vi "TEST STEER.vi"() -> ()   [LabVIEW 2023]
uses:
  ctrl defs/ctrl MOTOR SELECT.ctl
  <vilib>/Rock Robotics/WPI/ThirdParty/REV Robotics/REVLib/Typedef/Spark MAX Idle Mode.ctl
  ctrl defs/ctrl swerve motor.ctl
  ctrl defs/ctrl Spark MAX current limiting.ctl
  ctrl defs/ctrl motor PIDF coefficients.ctl
  <vilib>/Rock Robotics/WPI/ThirdParty/REV Robotics/REVLib/Typedef/Spark MAX Smart Motion Parameters.ctl
  <vilib>/Rock Robotics/WPI/MotorControl/WPI_MotorControlDeviceRef.ctl
  <vilib>/Rock Robotics/WPI/MotorControl/WPI_MotorControlType.ctl
  <vilib>/Rock Robotics/SystemInterfaces/DIO/FPGA_DIOPWMChannel.ctl
  <vilib>/Rock Robotics/WPI/PWM/WPI_PWMDeadband.ctl
  <vilib>/Rock Robotics/SystemInterfaces/DIO/FPGA_DIOChannel.ctl
  <vilib>/Rock Robotics/WPI/ThirdParty/Phoenix-LabVIEW/CANCoder/Controls/CTRE_Phoenix_CANcoder_DeviceRef.ctl
  <vilib>/Rock Robotics/WPI/ThirdParty/REV Robotics/REVLib/Typedef/Spark MAX Control Type.ctl
  Global INIT.vi
  <vilib>/Rock Robotics/WPI/ThirdParty/Phoenix-LabVIEW/CANCoder/Get/CTRE_Phoenix_CANcoder_GetSensorData.vi
panel:
  out "Absolute Position":dbl
  out "Velocity":dbl
  out "Position":dbl
  in  "Magnet Offset (Degrees)":dbl
  in  "Sensor Direction":bool
  in  "refnum name 2":string
  in  "CAN Bus":string
  in  "CAN ID 2":u8
  in  "Installed? 2":bool
  in  "description 2":string
  out "Sensor Velocity":dbl
  out "Sensor Position":dbl
  out "Hard Limit Rev":bool
  out "Hard Limit Fwd":bool
  in  "MOTOR %VBus":dbl(slide) scale=-1.0..1.0
  out "swerve STEER motors":T1[](array[typedef]) {"gear ratio" format="%_5f"; "MOTOR SELECT" items=["REV NEO"=5676, "REV NEO 550"=11000, "VEX Falcon"=6380, "WC Kraken"=6000]}
  in  "SAFETY":bool
  in  "commit to INIT":bool
  in  "commit WRITE":bool
  in  "Idle Mode":T3
  in  "Invert":bool
  in  "refnum name":string
  in  "CAN ID":u8
  in  "Installed?":bool
  in  "MOTOR SELECT":T2 items=["REV NEO"=5676, "REV NEO 550"=11000, "VEX Falcon"=6380, "WC Kraken"=6000]
  in  "description":string
  in  "stop":bool
  in  "Select\nSTEER motor":T7(ring)=enum."Front Left"
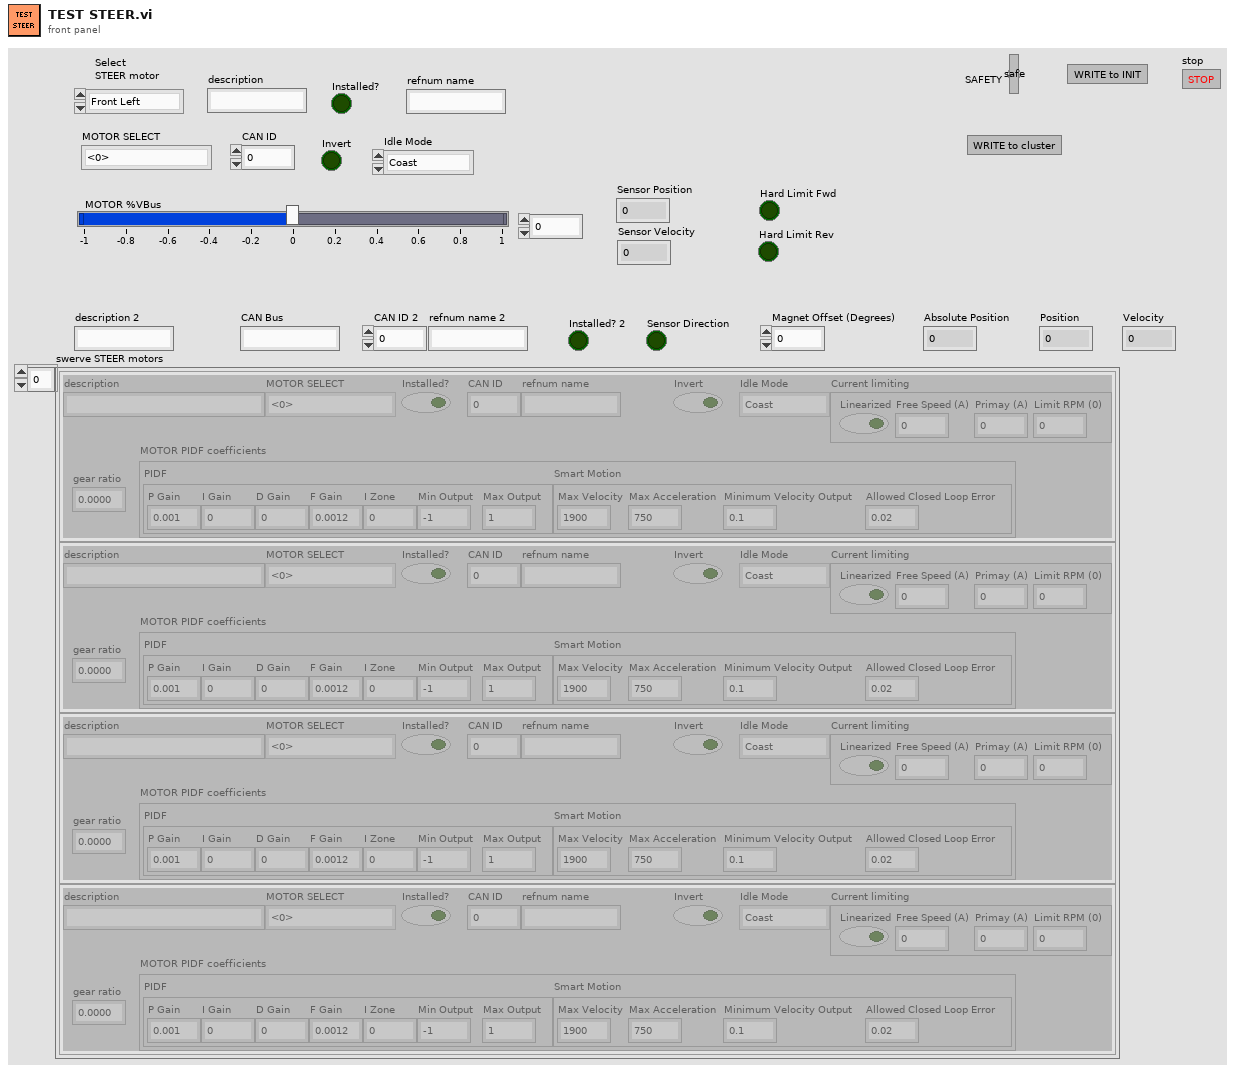
[diagram p1: front panel]
types:
  T1 = typedef "ctrl swerve motor.ctl" = cluster{"description":string, "MOTOR SELECT":T2, "Installed?":bool, "CAN ID":u8, "refnum name":string, "Invert":bool, "Idle Mode":T3, "Current limiting":T4, "MOTOR PIDF coefficients":T5, "gear ratio":dbl}
  T2 = typedef "ctrl MOTOR SELECT.ctl" = i16
  T3 = typedef "Spark MAX Idle Mode.ctl" = enum16{"Coast", "Brake"}
  T4 = typedef "ctrl Spark MAX current limiting.ctl" = cluster{"Linearized":bool, "Free Speed (A)":dbl, "Primay (A)":dbl, "Limit RPM (0)":u32}
  T5 = typedef "ctrl motor PIDF coefficients.ctl" = cluster{"PIDF":cluster{"P Gain":dbl, "I Gain":dbl, "D Gain":dbl, "F Gain":dbl, "I Zone":dbl, "Min Output":dbl, "Max Output":dbl}, "Smart Motion":T6}
  T6 = typedef "Spark MAX Smart Motion Parameters.ctl" = cluster{"Max Velocity":dbl, "Max Acceleration":dbl, "Minimum Velocity Output":dbl, "Allowed Closed Loop Error":dbl}
  T7 = enum16{"Front Right", "Front Left", "Rear Left", "Rear Right"}
  T8 = typedef "CTRE_Phoenix_CANcoder_DeviceRef.ctl" = cluster{"DeviceStatus":errorcluster, "Device Number":u8, "Handle":u64, "UsageFrame":u32, "Library Path":path}
  T9 = typedef "WPI_MotorControlDeviceRef.ctl" = cluster{"DeviceStatus":errorcluster, "Type":T10, "PWM":cluster{"PWM Channel":T11, "DeadBand":T12}, "CAN":cluster{"Device Number":u8, "SetOutput VI Ref":variant, "GetOutput VI Ref":variant, "Enable VI Ref":variant, "Disable VI Ref":variant, "Data":variant}, "Invert":bool, "DIO PWM":cluster{"PWM \"Enable\" Channel":T11, "DIOChannel":T13, "PWM Rate":dbl}}
  T10 = typedef "WPI_MotorControlType.ctl" = enum16{"PWM", "CAN", "DIO PWM"}
  T11 = typedef "FPGA_DIOPWMChannel.ctl" = enum8{"PWM 0", "PWM 1", "PWM 2", "PWM 3", "PWM 4", "PWM 5", "PWM 6", "PWM 7", "PWM 8", "PWM 9", "PWM MXP 0", "PWM MXP 1", "PWM MXP 2", "PWM MXP 3", "PWM MXP 4", "PWM MXP 5", "PWM MXP 6", "PWM MXP 7", "PWM MXP 8", "PWM MXP 9", "Invalid"}
  T12 = typedef "WPI_PWMDeadband.ctl" = cluster{"Name":string, "maxPositivePwm":i32, "minPositivePwm":i32, "centerPwm":i32, "maxNegativePwm":i32, "minNegativePwm":i32, "angularRange":u16}
  T13 = typedef "FPGA_DIOChannel.ctl" = enum8{"DIO 0", "DIO 1", "DIO 2", "DIO 3", "DIO 4", "DIO 5", "DIO 6", "DIO 7", "DIO 8", "DIO 9", "DIO MXP 0", "DIO MXP 1", "DIO MXP 2", "DIO MXP 3", "DIO MXP 4", "DIO MXP 5", "DIO MXP 6", "DIO MXP 7", "DIO MXP 8", "DIO MXP 9", "DIO MXP 10", "DIO MXP 11", "DIO MXP 12", "DIO MXP 13", "DIO MXP 14", "DIO MXP 15", "SPI Port CS1", "SPI Port CS2", "SPI Port CS3", "SPI Port MISO", "SPI Port MOSI", "Invalid"}
  T14 = typedef "ctrl CANcoder.ctl" = cluster{"description":string, "Installed?":bool, "CAN ID":u8, "CAN Bus":string, "refnum name":string, "Sensor Direction":bool, "Magnet Offset (Degrees)":dbl, "gear ratio":dbl}
  T15 = typedef "Spark MAX Control Type.ctl" = enum16{"Percent VBus", "Voltage", "Velocity", "Position", "Smart Motion", "Current", "Smart Velocity"}
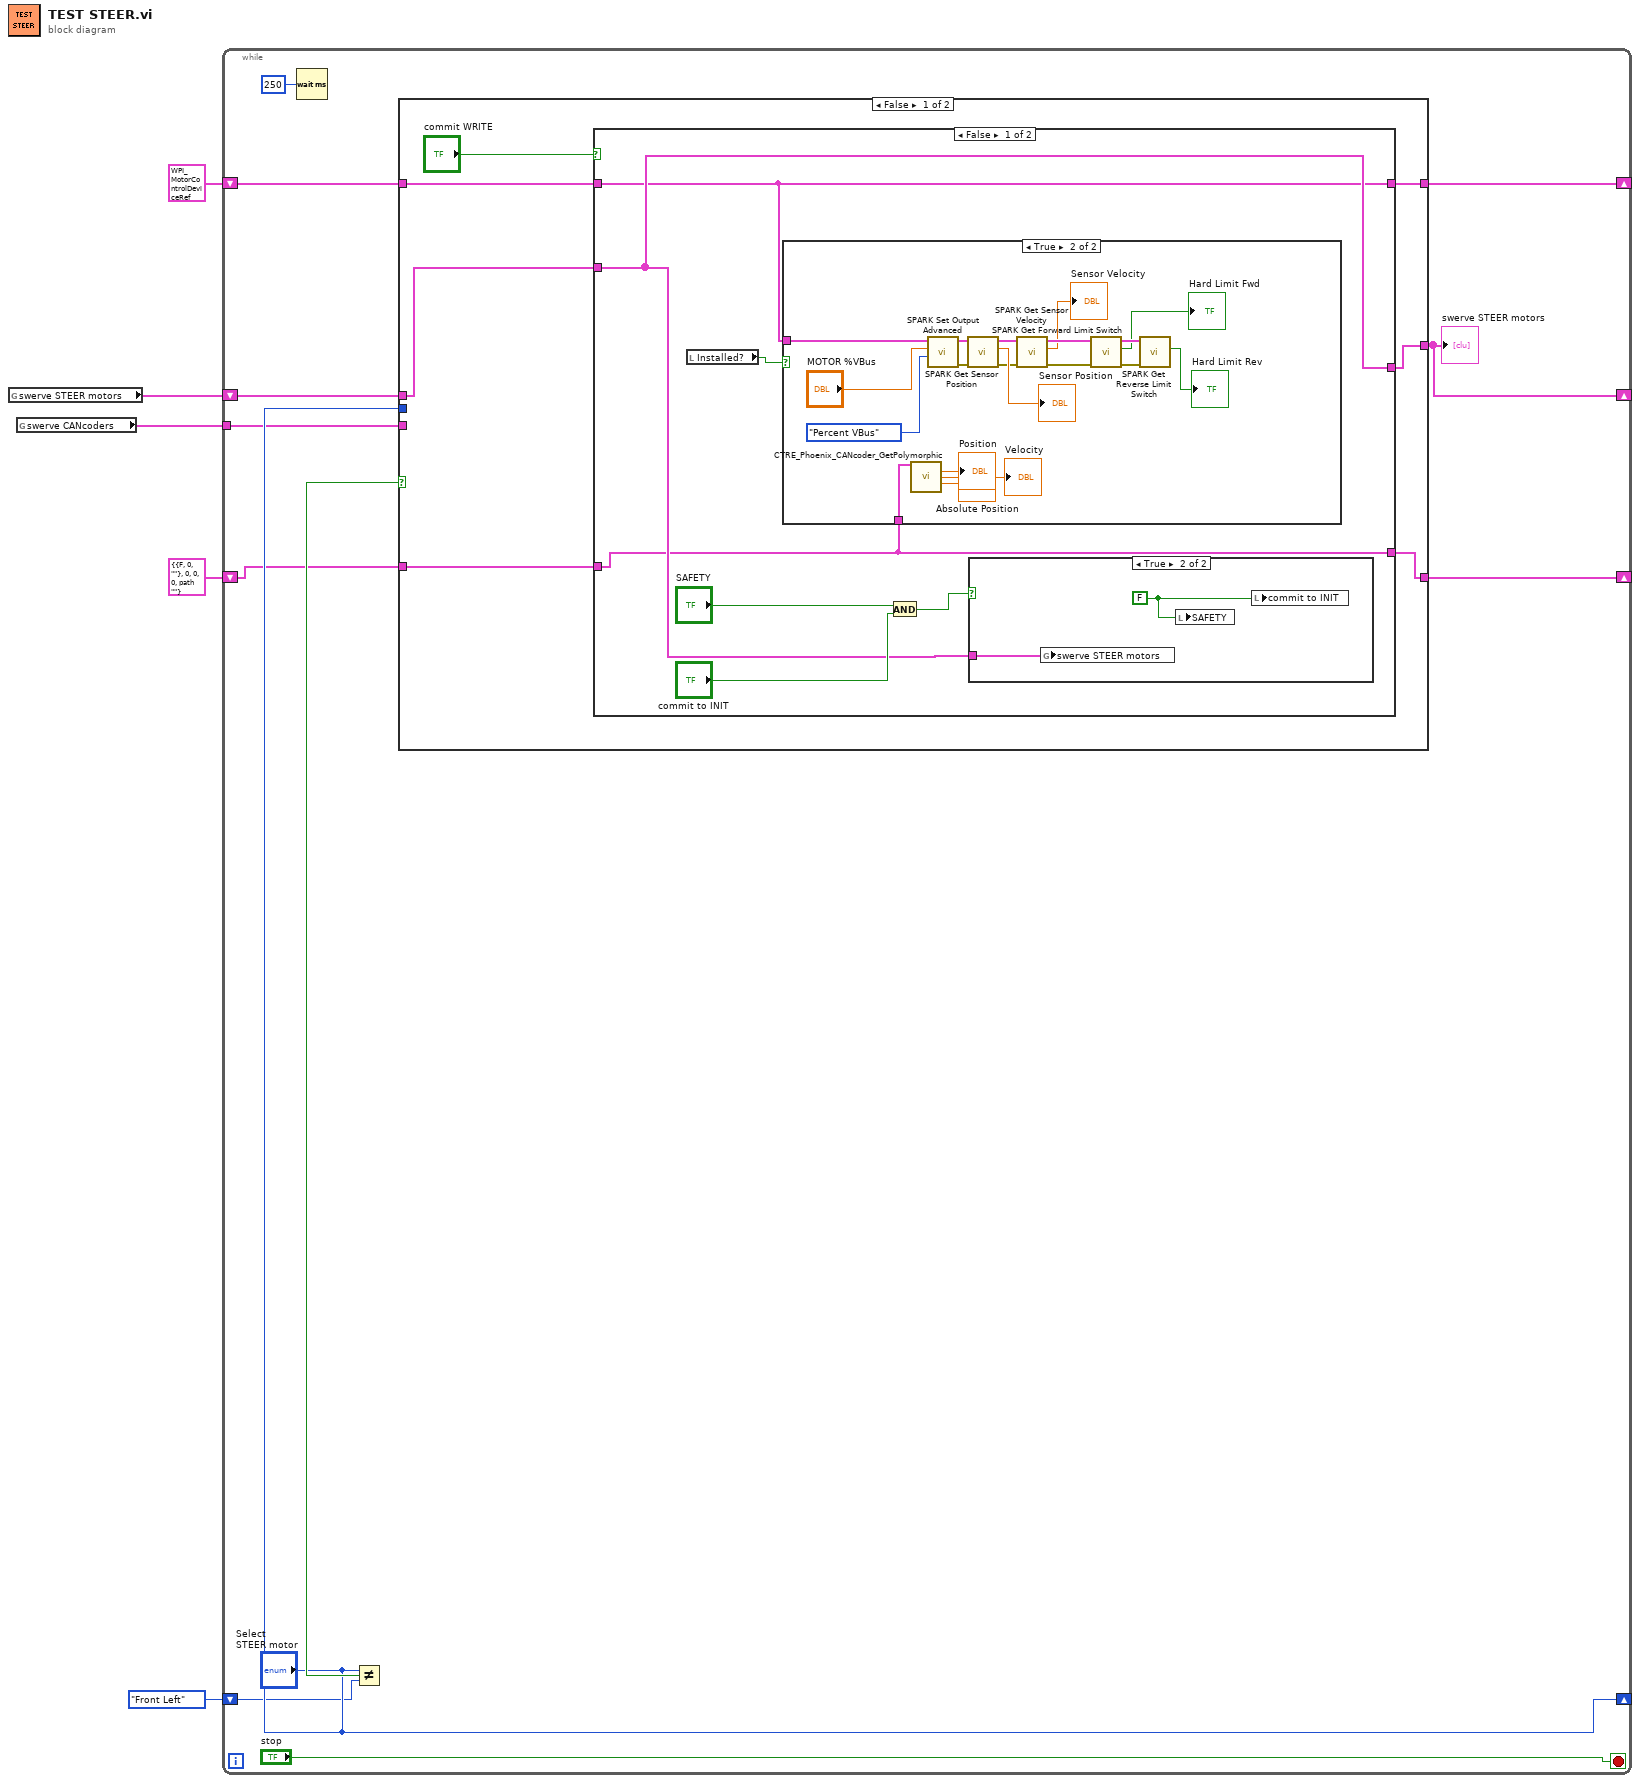
[diagram p0: block diagram]
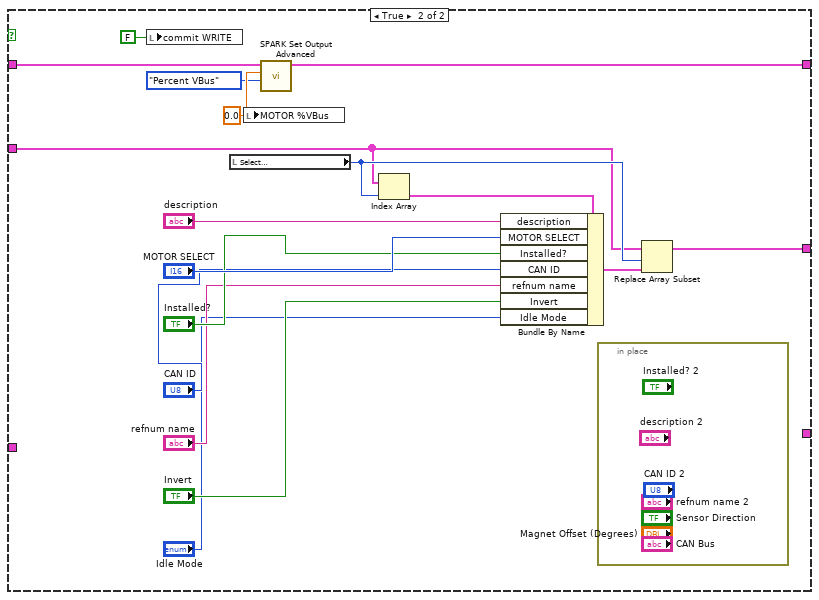
[diagram p4: hidden frame]
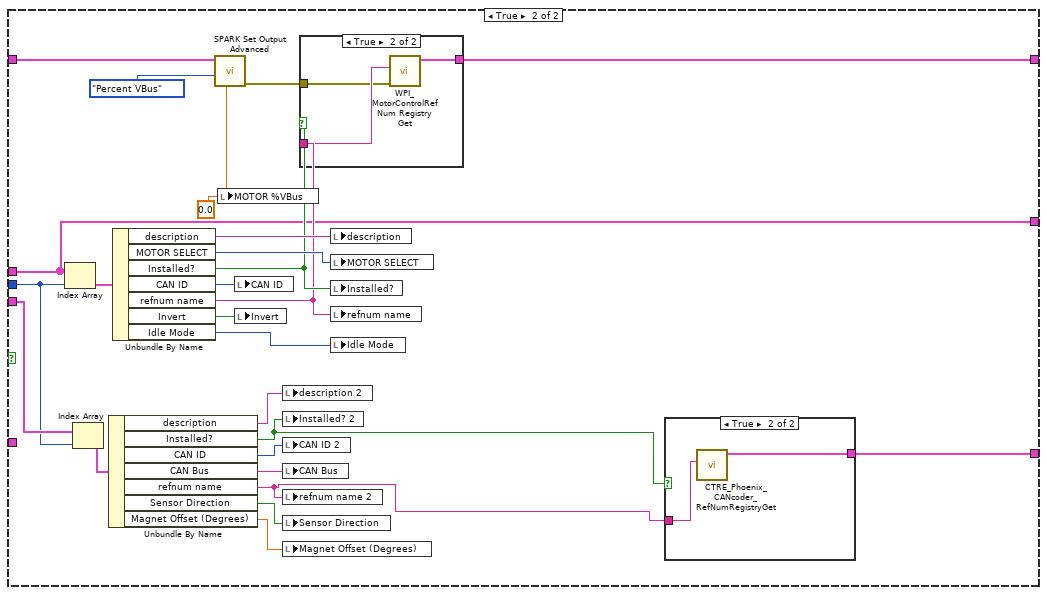
[diagram p5: hidden frame]
diagram:
  n1 = global read "Global INIT.vi" "swerve STEER motors"() -> (w5:T1[])
  n2 = global read "Global INIT.vi" "swerve CANcoders"() -> (w2:T14[])
  n3 = while {
    shift-right: ["Select\nSTEER motor"] -> _
    shift-left: T7."Front Left" ("Select\nSTEER motor") -> [w14]
    shift-right: [w12] -> _
    shift-left: w5 -> [w13]
    shift-right: [w10] -> _
    shift-left: T9 {"DeviceStatus"={"status"=FALSE, "code"=0, "source"=""}, "Type"=enum."PWM", "PWM"={"PWM Channel"=enum."Invalid", "DeadBand"={"Name"="", "maxPositivePwm"=0, "minPositivePwm"=0, "centerPwm"=0, "maxNegativePwm"=0, "minNegativePwm"=0, "angularRange"=0}}, "CAN"={"Device Number"=0, "SetOutput VI Ref"=variant, "GetOutput VI Ref"=variant, "Enable VI Ref"=variant, "Disable VI Ref"=variant, "Data"=variant}, "Invert"=FALSE, "DIO PWM"={"PWM \"Enable\" Channel"=enum."Invalid", "DIOChannel"=enum."Invalid", "PWM Rate"=0.0}} ("MotorControlDevRef") -> [w9]
    tunnel: w2 -> [w8]
    shift-right: [w7] -> _
    shift-left: T8 {"DeviceStatus"={"status"=FALSE, "code"=0, "source"=""}, "Device Number"=0, "Handle"=0, "UsageFrame"=0, "Library Path"=path ""} ("CTRE_CANcoder_DeviceRef") -> [w6]
    stop <- "stop" stop-if-true
    n4 = Wait (ms)(milliseconds to wait=u32 250) -> ()  [unwired: 1 out]
    n5 = Not Equal?(x="Select\nSTEER motor", y=w14) -> (x != y?=w16:bool)
    n6 = case shown="False" w16 {
      tunnel: w13 -> [w20 w81]
      tunnel: "Select\nSTEER motor" -> [_ w79]
      tunnel: [w23 w81] -> w12
      tunnel: [w21 w86] -> w10
      tunnel: w9 -> [w22 w83]
      tunnel: w8 -> [_ w80]
      tunnel: [w18 w77] -> w7
      tunnel: w6 -> [w19 _]
      frame False {
        n7 = case shown="False" "commit WRITE" {
          tunnel: w20 -> [w28 w66]
          tunnel: [w28 w68] -> w23
          tunnel: w22 -> [w25 w56]
          tunnel: [w25 w55] -> w21
          tunnel: w19 -> [w26 _]
          tunnel: [w26 _] -> w18
          frame False {
            n8 = local read "Installed?"() -> (w27:bool)
            n9 = case shown="True" w27 {
              tunnel: w25 -> [_ w50]
              tunnel: w26 -> [_ w35]
              frame False {
              }
              frame True {
                n10 = call-poly <vilib>:"CTRE_Phoenix_CANcoder_GetPolymorphic.vi"("CTRE_CANcoder_DeviceRef"=w35) -> ("Position"=→"Position":dbl, "Velocity"=→"Velocity":dbl, "Absolute Position"=→"Absolute Position":dbl)  [unwired: 10 in, 2 out]
                n11 = call <vilib>:"SPARK Set Output Advanced.vi"("Control Mode"=Spark_MAX_Control_Type."Percent VBus", "Setpoint"="MOTOR %VBus", "MotorControlDevRef"=w50) -> ("error out"=w40:errorcluster, "MotorControlDevRef"=w41:T9)  [unwired: 7 in]
                n12 = call <vilib>:"SPARK Get Sensor Position.vi"("error in (no error)"=w40, "MotorControlDevRef in"=w41) -> ("error out"=w43:errorcluster, "Sensor Position"=→"Sensor Position":dbl, "MotorControlDevRef out"=w47:T9)  [unwired: 6 in, 1 out]
                n13 = call <vilib>:"SPARK Get Sensor Velocity.vi"("error in (no error)"=w43, "MotorControlDevRef in"=w47) -> ("error out"=w42:errorcluster, "Sensor Velocity"=→"Sensor Velocity":dbl, "MotorControlDevRef out"=w46:T9)  [unwired: 6 in, 1 out]
                n14 = call <vilib>:"SPARK Get Forward Limit Switch.vi"("error in (no error)"=w42, "MotorControlDevRef in"=w46) -> ("error out"=w36:errorcluster, "Hard Limit Fwd"=→"Hard Limit Fwd":bool, "MotorControlDevRef out"=w39:T9)  [unwired: 6 in, 1 out]
                n15 = call <vilib>:"SPARK Get Reverse Limit Switch.vi"("error in (no error)"=w36, "MotorControlDevRef in"=w39) -> ("Hard Limit Rev"=→"Hard Limit Rev":bool)  [unwired: 6 in, 3 out]
              }
            }
            n16 = And(x="SAFETY", y="commit to INIT") -> (x .and. y?=w29:bool)
            n17 = case shown="True" w29 {
              tunnel: w28 -> [_ w52]
              frame False {
              }
              frame True {
                w51 = FALSE ("SAFETY")
                n18 = global write "Global INIT.vi" "swerve STEER motors"(w52) -> ()
                n19 = local write "SAFETY"(w51) -> ()
                n20 = local write "commit to INIT"(w51) -> ()
              }
            }
          }
          frame True {
            w54 = 0.0 ("Setpoint")
            n21 = local write "commit WRITE"(FALSE ("commit WRITE")) -> ()
            n22 = local read "Select\nSTEER motor"() -> (w67:T7)
            n23 = local write "MOTOR %VBus"(w54) -> ()
            n24 = call <vilib>:"SPARK Set Output Advanced.vi"("Control Mode"=Spark_MAX_Control_Type."Percent VBus", "Setpoint"=w54, "MotorControlDevRef"=w56) -> ("MotorControlDevRef"=w55:T9)  [unwired: 7 in, 1 out]
            n25 = Index Array(array=w66, index=w67) -> (element=w65:T1)
            n26 = Bundle By Name(cluster=w65, "description"="description", "MOTOR SELECT"="MOTOR SELECT", "Installed?"="Installed?", "CAN ID"="CAN ID", "refnum name"="refnum name", "Invert"="Invert", "Idle Mode"="Idle Mode") -> (w64:T1)
            n27 = in-place {
            }
            n28 = Replace Array Subset(array=w66, new element=w64, index=w67) -> (w68:T1[])
          }
        }
      }
      frame True {
        w85 = 0.0 ("Setpoint")
        n29 = Index Array(array=w81, index=w79) -> (element=w94:T1)
        n30 = Index Array(array=w80, index=w79) -> (element=w78:T14)
        n31 = Unbundle By Name(w78) -> ("description"=w76:string, "Installed?"=w71:bool, "CAN ID"=w73:u8, "CAN Bus"=w74:string, "refnum name"=w70:string, "Sensor Direction"=w75:bool, "Magnet Offset (Degrees)"=w72:dbl)
        n32 = Unbundle By Name(w94) -> ("description"=w93:string, "MOTOR SELECT"=w91:T2, "Installed?"=w88:bool, "CAN ID"=w89:u8, "refnum name"=w87:string, "Invert"=w90:bool, "Idle Mode"=w92:T3)
        n33 = call <vilib>:"SPARK Set Output Advanced.vi"("Control Mode"=Spark_MAX_Control_Type."Percent VBus", "Setpoint"=w85, "MotorControlDevRef"=w83) -> ("error out"=w82:errorcluster)  [unwired: 7 in, 1 out]
        n34 = local write "MOTOR %VBus"(w85) -> ()
        n35 = local write "CAN ID"(w89) -> ()
        n36 = local write "Invert"(w90) -> ()
        n37 = local write "description 2"(w76) -> ()
        n38 = local write "Installed? 2"(w71) -> ()
        n39 = local write "CAN ID 2"(w73) -> ()
        n40 = local write "CAN Bus"(w74) -> ()
        n41 = local write "refnum name 2"(w70) -> ()
        n42 = local write "Sensor Direction"(w75) -> ()
        n43 = local write "Magnet Offset (Degrees)"(w72) -> ()
        n44 = case shown="True" w88 {
          tunnel: w87 -> [_ w99]
          tunnel: [_ w98] -> w86
          tunnel: w82 -> [_ w97]
          frame False {
          }
          frame True {
            n45 = call <vilib>:"WPI_MotorControlRefNum Registry Get.vi"("error in (no error)"=w97, "refnum name"=w99) -> ("MotorControlDevRef"=w98:T9)  [unwired: 8 in, 1 out]
          }
        }
        n46 = local write "description"(w93) -> ()
        n47 = local write "MOTOR SELECT"(w91) -> ()
        n48 = local write "Installed?"(w88) -> ()
        n49 = local write "refnum name"(w87) -> ()
        n50 = local write "Idle Mode"(w92) -> ()
        n51 = case shown="True" w71 {
          tunnel: w70 -> [_ w96]
          tunnel: [_ w95] -> w77
          frame False {
          }
          frame True {
            n52 = call <vilib>:"CTRE_Phoenix_CANcoder_RefNumRegistryGet.vi"("refnum name"=w96) -> ("CTRE_CANcoder_DeviceRef"=w95:T8)  [unwired: 9 in, 1 out]
          }
        }
      }
    }
    "swerve STEER motors" <- w12
  }
